vi "Set Letter.vi"(10 "letter":string, 11 "Letter in (new)":refnum<class "Letter.lvclass">) -> (3 "Letter out":refnum<class "Letter.lvclass">)   [LabVIEW 2015, in "Letter.lvclass"]
uses:
  Letter.lvclass
  Letter.lvclass/Letter.ctl
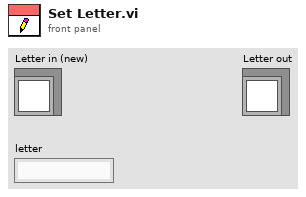
[diagram p1: front panel]
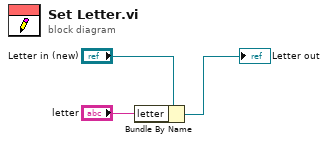
[diagram p0: block diagram]
diagram:
  n1 = Bundle By Name(cluster="Letter in (new)", "letter"="letter") -> (→"Letter out":refnum<class "Letter.lvclass">)
